vi "Launcher.vi"() -> ()   [LabVIEW 2022 SP3]
doc: "JKI State Machine Objects (SMO) 1.0.0.5\nJKI - JKI\nCopyright (c) 2016, JKI"
uses:
  002_SRC/Splashy/Splashy.lvclass
  C:/Program Files (x86)/National Instruments/LabVIEW 2022/vi.lib/JKI/JKI SMO/SMO/SMO.lvclass
  C:/Program Files (x86)/National Instruments/LabVIEW 2022/vi.lib/JKI/JKI SMO/SMO.UI/SMO.UI.lvclass
  002_SRC/GUI/GUI.lvclass
  <vilib>/JKI/JKI SMO/SMO/SMO.lvclass/SMO.ctl
  <vilib>/JKI/JKI SMO/SMO.UI/SMO.UI.lvclass/SMO.UI.ctl
  <vilib>/JKI/JKI SMO/SMO/Typedefs/SMOState --Enum.ctl
  f04c7903-df52-4a90-82d6-ebb4e2f21dec.vi
  <vilib>/JKI/JKI SMO/SMO/Private/ReftoDVR--SMO.vi
  <vilib>/JKI/JKI SMO/SMO.UI/SMO.UI.ReftoDVR.vi
  <vilib>/JKI/JKI SMO/SMO/SMO.lvclass
  <vilib>/JKI/JKI SMO/SMO.UI/SMO.UI.lvclass
  D:/DSUsers/uib01493/000_SD_Card/009_Projects/CIS_580/SReTT_GUI/002_SRC/Splashy/Splashy.lvclass
  D:/DSUsers/uib01493/000_SD_Card/009_Projects/CIS_580/SReTT_GUI/002_SRC/GUI/GUI.lvclass
  4c252a11-53c5-4d78-9af7-4f6c26702880.vi
panel:
  out "error out":errorcluster
  in  "Stop":bool
  # "SMO Splash Test Launcher"
  # "For instructions on how to use the JKI State Machine Objects, examples and video tutorials, visit:\nhttp://jki.net/state-machine-objects/\n\nJKI State Machine Objects™\nhttp://jki.net/state-machine-objects/\nCopyright (C) 2005-2015, JKI <info@jki.net>\nALL RIGHTS RESERVED"
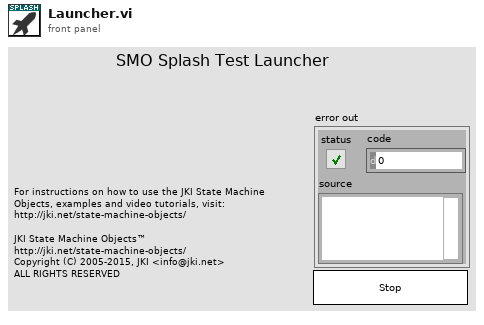
[diagram p1: front panel]
types:
  T1 = enum32{"Invalid", "Standard", "Closed", "Hidden", "Minimized", "Maximized"}
  T2 = typedef "SMO.lvclass/Public Events.ctl" = cluster{"Error":refnum<user-event>, "State":refnum<user-event>, "Reserve State":refnum<user-event>}
  T3 = typedef "SMO.UI.lvclass/PublicEvents--Cluster.ctl" = cluster{"UI Hidden":refnum<user-event>, "UI State":refnum<user-event>}
  T4 = typedef "SMO.lvclass/SMOState --Enum.ctl" = enum16{"unknown", "Created", "Started", "Stopped"}
  T5 = typedef "GUI.lvclass/PublicEvents--Cluster.ctl" = cluster{"Value Changed":refnum<user-event>}
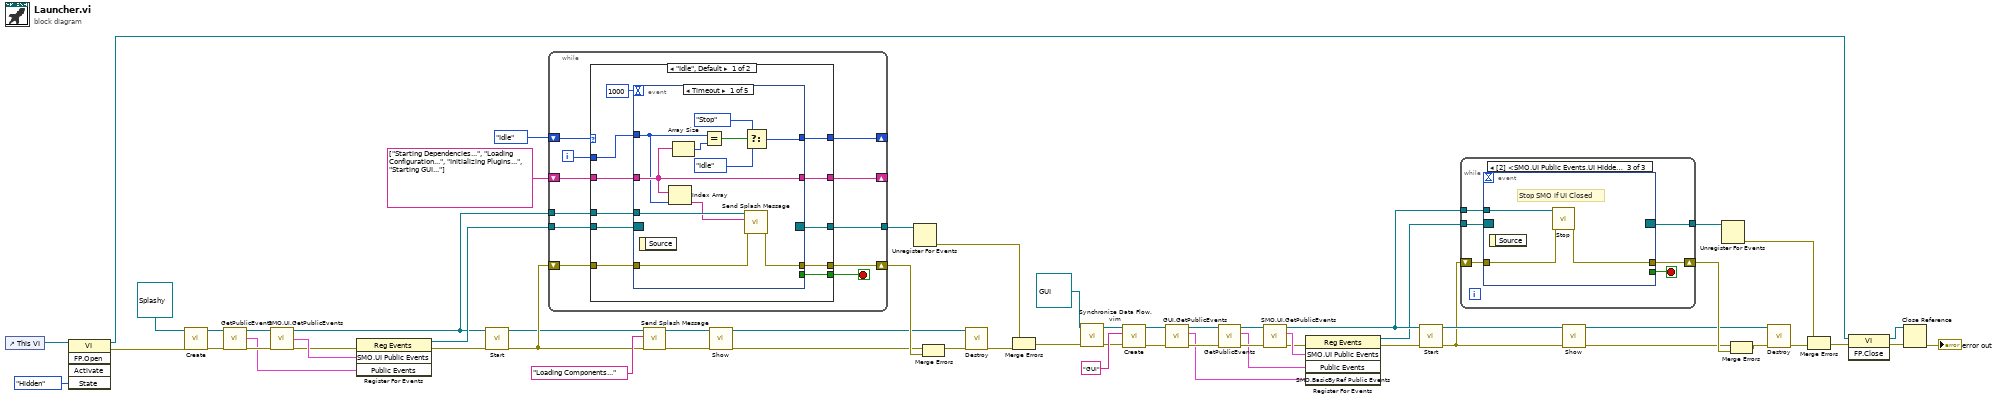
[diagram p0: block diagram]
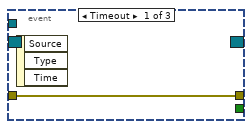
[diagram p2: hidden frame]
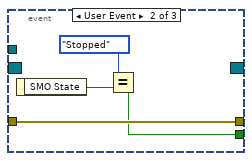
[diagram p3: hidden frame]
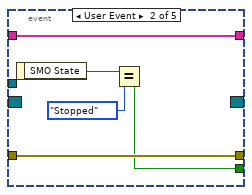
[diagram p4: hidden frame]
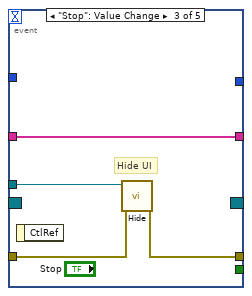
[diagram p5: hidden frame]
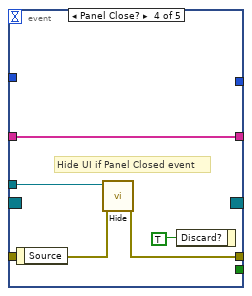
[diagram p6: hidden frame]
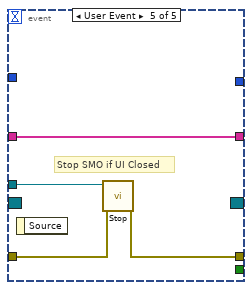
[diagram p7: hidden frame]
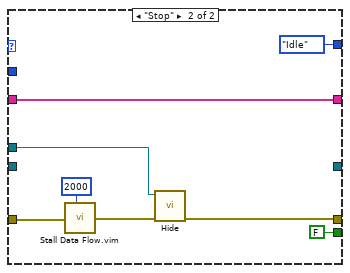
[diagram p8: hidden frame]
diagram:
  n1 = control-ref of="This VI"() -> (w32:refnum<vi>)
  n2 = invoke class="VI" method="FP.Open"(reference=w32, "State"=T1."Hidden") -> (reference out=w29:refnum<vi>, error out=w37:errorcluster)  [unwired: 3 in, 3 out]
  n3 = call <vilib>:"Create.vi"("error in (no error)"=w37, "SMO"=refnum<class "Splashy.lvclass"> refnum ("SMO.Template.lvclass")) -> ("error out"=w43:errorcluster, "SMO out"=w45:refnum<class "Splashy.lvclass">)  [unwired: 7 in, 1 out]
  n4 = call <vilib>:"GetPublicEvents.vi"("error in (no error)"=w43, "SMO"=w45) -> ("error out"=w42:errorcluster, "Public Events"=w41:T2, "SMO out"=w44:refnum<class "Splashy.lvclass">)  [unwired: 7 in]
  n5 = call <vilib>:"SMO.UI.GetPublicEvents.vi"("error in (no error)"=w42, "SMO.UI"=w44) -> ("error out"=w47:errorcluster, "SMO.UI Public Events"=w48:T3, "SMO.UI out"=w39:refnum<class "Splashy.lvclass">)  [unwired: 7 in]
  n6 = register-events(error in=w47, w48, w41) -> (reference out=w40:refnum<event-registration>, error out=w46:errorcluster)  [unwired: 1 in]
  n7 = call <vilib>:"Start.vi"("error in (no error)"=w46, "SMO"=w39) -> ("error out"=w52:errorcluster, "SMO out"=w49:refnum<class "Splashy.lvclass">)  [unwired: 8 in]
  n8 = while {
    shift-right: [w70] -> w59
    shift-left: w52 -> [w69]
    tunnel: w40 -> [w68]
    tunnel: [w67] -> w60
    tunnel: w39 -> [w66]
    shift-right: [w63] -> _
    shift-left: string[] ["Starting Dependencies...", "Loading Configuration...", "Initializing Plugins...", "Starting GUI..."] -> [w64]
    shift-right: [w62] -> _
    shift-left: enum16{"Idle", "Stop"}."Idle" -> [w61]
    i -> [w65]
    stop <- w71 stop-if-true
    n9 = case shown="\"Idle\", Default" w61 {
      tunnel: [w82 FALSE] -> w71
      tunnel: [w81 w112] -> w70
      tunnel: w69 -> [w80 w117]
      tunnel: w68 -> [w79 _]
      tunnel: [w78 _] -> w67
      tunnel: w66 -> [w77 w113]
      tunnel: w65 -> [w75 _]
      tunnel: w64 -> [w74 w118]
      tunnel: [w73 w118] -> w63
      tunnel: [w72 enum16{"Idle", "Stop"}."Idle"] -> w62
      frame "Idle", Default {
        n10 = event shown="[0] Timeout" {
          selector: w79 -> [_ _ _ _ _]
          dyn-events: [_ _ _ _ _] -> w78
          timeout: 1000 -> [_ _ _ _ _]
          tunnel: [_ w95 _ _ _] -> w82
          tunnel: w77 -> [w93 _ w102 w106 w111]
          tunnel: [w90 w98 w100 w104 w110] -> w81
          tunnel: w80 -> [w91 w98 w101 w105 w109]
          tunnel: w75 -> [w83 _ _ _ _]
          tunnel: w74 -> [w87 w94 w99 w103 w108]
          tunnel: [w87 w94 w99 w103 w108] -> w73
          tunnel: [w86 _ _ _ _] -> w72
          event Timeout {
            n11 = event-data() -> ()  [unwired: 1 in, 1 out]
            n12 = Index Array(array=w87, index=w83) -> (element=w92:string)
            n13 = Array Size(array=w87) -> (size(s)=w89:i32)
            n14 = Equal?(x=w83, y=w89) -> (x = y?=w88:bool)
            n15 = call-dynamic "Send Splash Message.vi"("error in (no error)"=w91, "Message"=w92, "Splashy"=w93) -> ("error out"=w90:errorcluster)  [unwired: 7 in, 1 out]
            n16 = Select(t=enum16{"Idle", "Stop"}."Stop", s=w88, f=enum16{"Idle", "Stop"}."Idle") -> (s? t:f=w86:enum16{"Idle", "Stop"})
          }
          event User Event {
            n17 = event-data() -> ("SMO State"=w97:T4)  [unwired: 1 in]
            n18 = Equal?(x=w97, y=SMOState_--Enum."Stopped") -> (x = y?=w95:bool)
          }
          event "Stop": Value Change {
            # "Hide UI"
            n19 = event-data() -> ()  [unwired: 1 in, 1 out]
            n20 = call <vilib>:"Hide.vi"("error in (no error)"=w101, "SMO.UI"=w102) -> ("error out"=w100:errorcluster)  [unwired: 8 in, 1 out]
          }
          event Panel Close? {
            # "Hide UI if Panel Closed event"
            n21 = event-data() -> ()  [unwired: 1 in, 1 out]
            n22 = call <vilib>:"Hide.vi"("error in (no error)"=w105, "SMO.UI"=w106) -> ("error out"=w104:errorcluster)  [unwired: 8 in, 1 out]
            n23 = event-data("Discard?"=TRUE ("OK")) -> ()  [unwired: 1 in, 1 out]
          }
          event User Event {
            # "Stop SMO if UI Closed"
            n24 = event-data() -> ()  [unwired: 1 in, 1 out]
            n25 = call <vilib>:"Stop.vi"("error in (no error)"=w109, "SMO"=w111) -> ("error out"=w110:errorcluster)  [unwired: 8 in, 1 out]
          }
        }
      }
      frame "Stop" {
        n26 = call "Stall Data Flow.vim"("value in"=w117, "milliseconds to wait"=u32 2000) -> ("value out"=w114:errorcluster)  [unwired: 1 out]
        n27 = call <vilib>:"Hide.vi"("error in (no error)"=w114, "SMO.UI"=w113) -> ("error out"=w112:errorcluster)  [unwired: 8 in, 1 out]
      }
    }
  }
  n28 = call-dynamic "Send Splash Message.vi"("error in (no error)"=w52, "Message"="Loading Components...", "Splashy"=w49) -> ("error out"=w51:errorcluster, "Splashy out"=w50:refnum<class "Splashy.lvclass">)  [unwired: 7 in]
  n29 = call <vilib>:"Show.vi"("error in (no error)"=w51, "SMO.UI"=w50) -> ("error out"=w56:errorcluster, "SMO.UI out"=w55:refnum<class "Splashy.lvclass">)  [unwired: 8 in]
  n30 = Unregister For Events(event registration refnum=w60) -> (error out=w58:errorcluster)  [unwired: 1 in]
  n31 = Merge Errors(w56, w59) -> (w54:errorcluster)
  n32 = call <vilib>:"Destroy.vi"("error in (no error)"=w54, "SMO"=w55) -> ("error out"=w35:errorcluster)  [unwired: 9 in]
  n33 = Merge Errors(w58, w35) -> (w2:errorcluster)
  n34 = call "Synchronize Data Flow.vim"("input 4"=w2, "input 1"=refnum<class "GUI.lvclass"> refnum ("GUI.lvclass")) -> ("output 4"=w1:errorcluster, "output 1"=w3:refnum<class "GUI.lvclass">)  [unwired: 2 in, 2 out]
  n35 = call <vilib>:"Create.vi"("error in (no error)"=w1, "Subsystem Name (optional)"="GUI", "SMO"=w3) -> ("error out"=w11:errorcluster, "SMO out"=w12:refnum<class "GUI.lvclass">)  [unwired: 6 in, 1 out]
  n36 = call "GUI.GetPublicEvents.vi"("error in (no error)"=w11, "GUI"=w12) -> ("error out"=w10:errorcluster, "SMO.BasicByRef Public Events"=w8:T5, "GUI out"=w9:refnum<class "GUI.lvclass">)  [unwired: 7 in]
  n37 = call <vilib>:"GetPublicEvents.vi"("error in (no error)"=w10, "SMO"=w9) -> ("error out"=w19:errorcluster, "Public Events"=w18:T2, "SMO out"=w7:refnum<class "GUI.lvclass">)  [unwired: 7 in]
  n38 = call <vilib>:"SMO.UI.GetPublicEvents.vi"("error in (no error)"=w19, "SMO.UI"=w7) -> ("error out"=w22:errorcluster, "SMO.UI Public Events"=w23:T3, "SMO.UI out"=w21:refnum<class "GUI.lvclass">)  [unwired: 7 in]
  n39 = register-events(error in=w22, w23, w18, w8) -> (reference out=w17:refnum<event-registration>, error out=w20:errorcluster)  [unwired: 1 in]
  n40 = call <vilib>:"Start.vi"("error in (no error)"=w20, "SMO"=w21) -> ("error out"=w13:errorcluster, "SMO out"=w14:refnum<class "GUI.lvclass">)  [unwired: 8 in]
  n41 = while {
    shift-right: [w124] -> w27
    shift-left: w13 -> [w123]
    tunnel: w17 -> [w122]
    tunnel: [w121] -> w28
    tunnel: w21 -> [w120]
    stop <- w125 stop-if-true
    n42 = event shown="[2] <SMO.UI Public Events.UI Hidden>: User Event" {
      selector: w122 -> [_ _ _]
      dyn-events: [_ _ _] -> w121
      timeout: _ -> [_ _ _]
      tunnel: [_ w127 _] -> w125
      tunnel: w120 -> [_ _ w133]
      tunnel: [w126 w130 w132] -> w124
      tunnel: w123 -> [w126 w130 w131]
      event Timeout {
        n43 = event-data() -> ()  [unwired: 1 in, 3 out]
      }
      event User Event {
        n44 = event-data() -> ("SMO State"=w129:T4)  [unwired: 1 in]
        n45 = Equal?(x=SMOState_--Enum."Stopped", y=w129) -> (x = y?=w127:bool)
      }
      event User Event {
        # "Stop SMO if UI Closed"
        n46 = event-data() -> ()  [unwired: 1 in, 1 out]
        n47 = call <vilib>:"Stop.vi"("error in (no error)"=w131, "SMO"=w133) -> ("error out"=w132:errorcluster)  [unwired: 8 in, 1 out]
      }
    }
  }
  n48 = call <vilib>:"Show.vi"("error in (no error)"=w13, "SMO.UI"=w14) -> ("error out"=w24:errorcluster, "SMO.UI out"=w15:refnum<class "GUI.lvclass">)  [unwired: 8 in]
  n49 = Unregister For Events(event registration refnum=w28) -> (error out=w26:errorcluster)  [unwired: 1 in]
  n50 = Merge Errors(w24, w27) -> (w16:errorcluster)
  n51 = call <vilib>:"Destroy.vi"("error in (no error)"=w16, "SMO"=w15) -> ("error out"=w25:errorcluster)  [unwired: 9 in]
  n52 = Merge Errors(w26, w25) -> (w6:errorcluster)
  n53 = invoke class="VI" method="FP.Close"(reference=w29, error in=w6) -> (reference out=w34:refnum<vi>, error out=w33:errorcluster)  [unwired: 1 in, 1 out]
  n54 = Close Reference(reference=w34, error in (no error)=w33) -> (error out=→"error out":errorcluster)
